vi "PathFinder.vi"(7 "All Lines":T3, 8 "Target Z":dbl format="%#_13g", 9 "Target X":dbl format="%#_13g", 11 "Posit Array":T1[](array[typedef])) -> (0 "Same Line +Dir?":bool, 1 "Path Found?":bool, 2 "Next Pos":cluster{"Line Index":i32, "Line Pos Index ":i32}, 3 "Shortest Path":T2[](array[typedef]), 4 "Index on Line":i32)   [LabVIEW 2014, in "Map Data.lvlib"]
uses:
  Map Data.lvlib
  All-Lines.ctl
  LineCluster.ctl
  LineConnection.ctl
  Components/PathFinder/Controls/PathControl.ctl
  Contact Data/Position.ctl
  Contact Data/Contact Data.lvlib
panel:
  out "All Distances":i32[](array[numeric])
  out "Distance (Points)":i32
  out "Path taken out":T2[][](array[typedef])
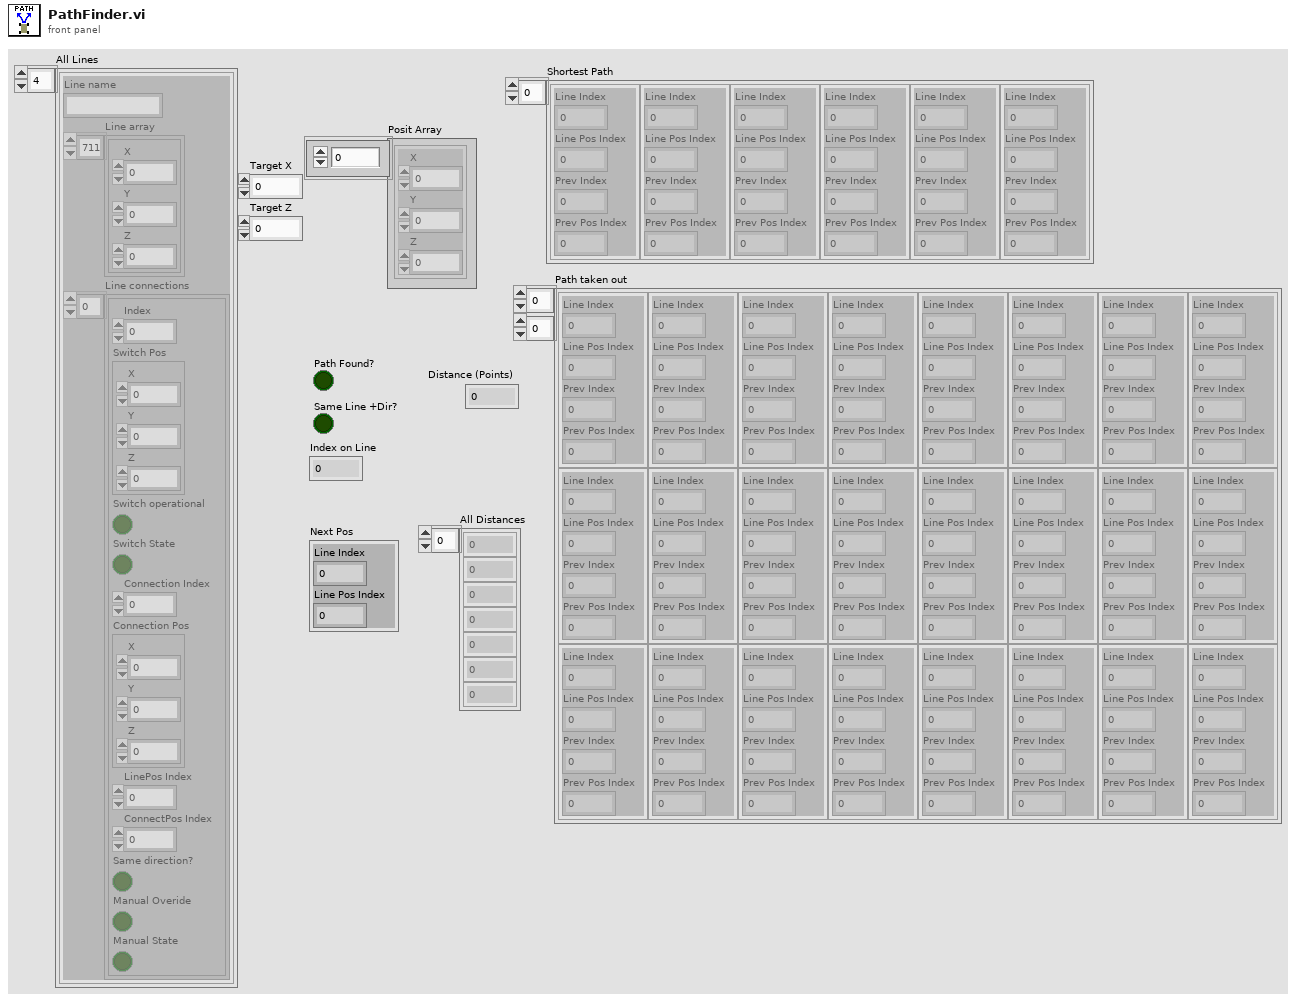
[diagram p1: front panel]
types:
  T1 = typedef "Contact Data.lvlib/Position.ctl" = cluster{"X":dbl, "Y":dbl, "Z":dbl}
  T2 = typedef "PathControl.ctl" = cluster{"Line Index":i32, "Line Pos Index ":i32, "Prev Index ":i32, "Prev Pos Index":i32}
  T3 = typedef "Map Data.lvlib/All-Lines.ctl" = T4[]
  T4 = typedef "Map Data.lvlib/LineCluster.ctl" = cluster{"Line name":string, "Line array":cluster{"X":dbl, "Y":dbl, "Z":dbl}[], "Line connections":T5[]}
  T5 = typedef "LineConnection.ctl" = cluster{"Index":i32, "Switch Pos":cluster{"X":dbl, "Y":dbl, "Z":dbl}, "Switch operational":bool, "Switch State":bool, "Connection Index":i32, "Connection Pos":cluster{"X":dbl, "Y":dbl, "Z":dbl}, "LinePos Index":i32, "ConnectPos Index":i32, "Same direction?":bool, "Manual Overide":bool, "Manual State":bool}
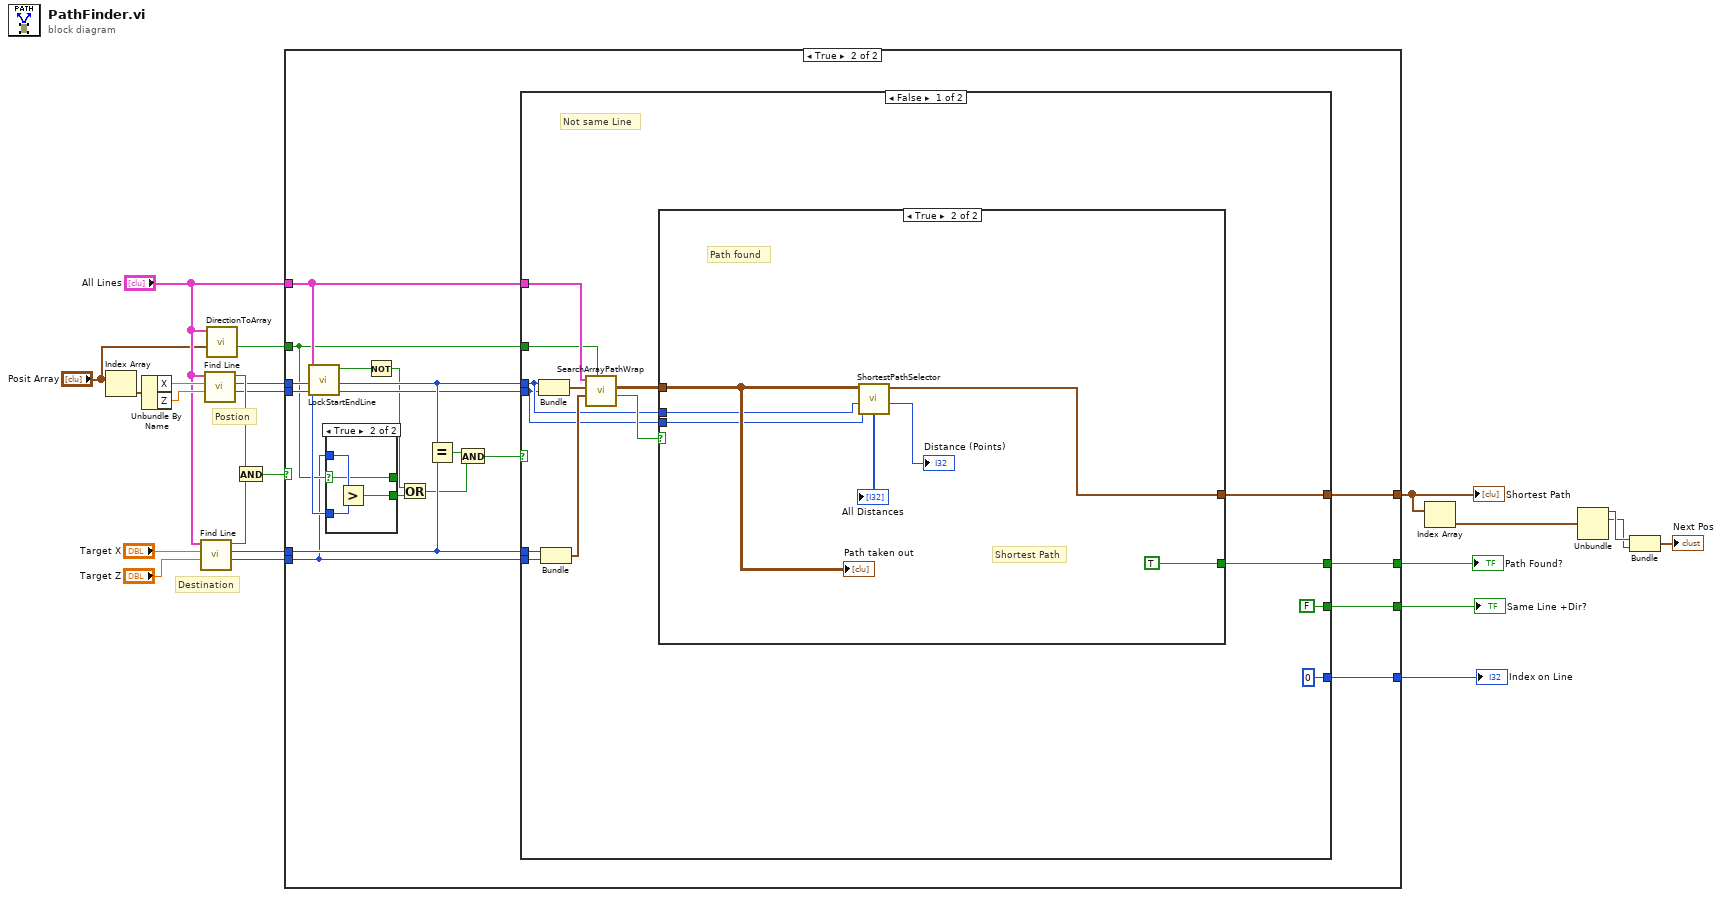
[diagram p0: block diagram]
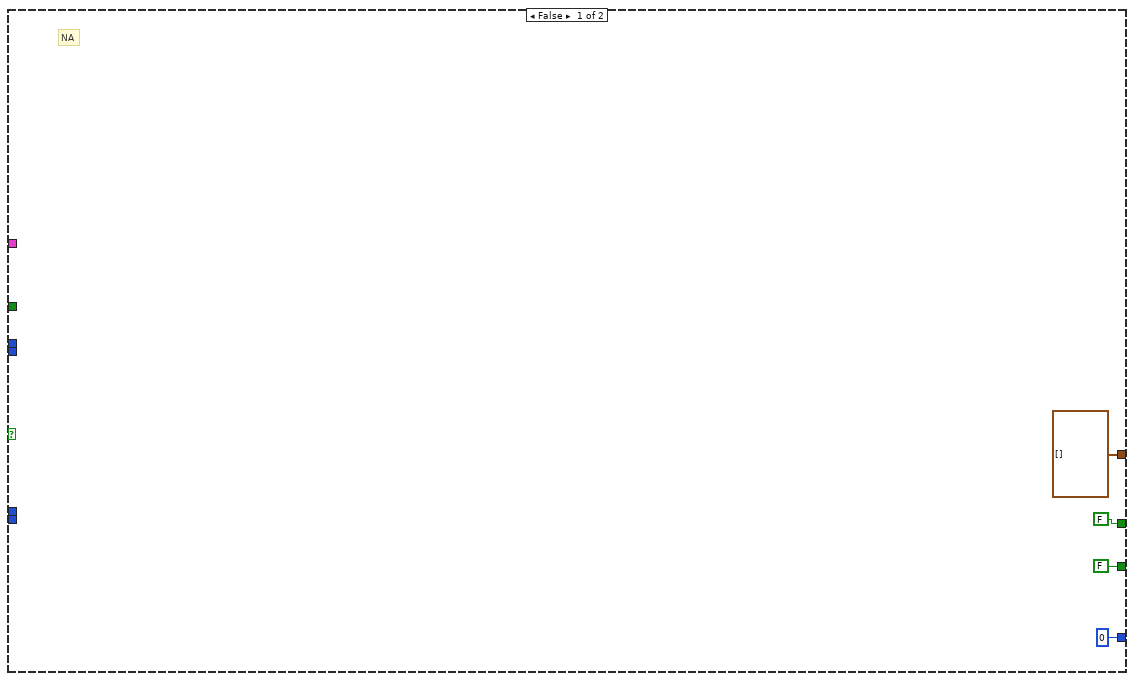
[diagram p2: hidden frame]
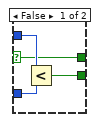
[diagram p3: hidden frame]
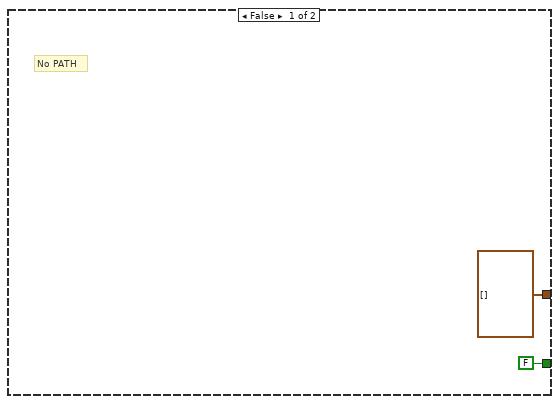
[diagram p4: hidden frame]
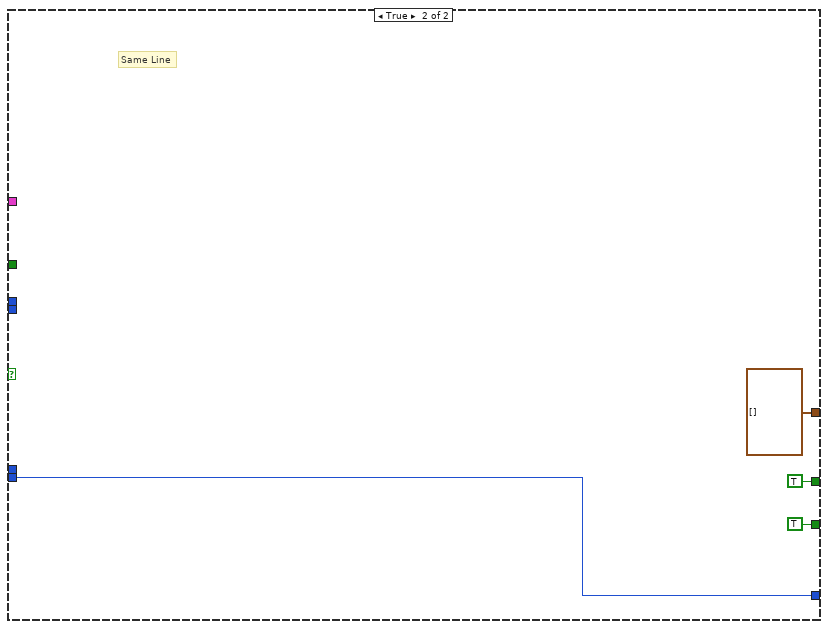
[diagram p5: hidden frame]
diagram:
  # "Postion"
  # "Destination"
  n1 = Index Array(array="Posit Array") -> (element=w10:T1)  [unwired: 1 in]
  n2 = Unbundle By Name(w10) -> ("X"=w9:dbl, "Z"=w8:dbl)
  n3 = call "Find Line.vi"("Z"="Target Z", "X"="Target X", "All Lines"="All Lines") -> ("Index on Line"=w15:i32, "Nearest Line"=w16:i32, "Line found?"=w21:bool)  [unwired: 5 in, 1 out]
  n4 = call "Find Line.vi"("Z"=w8, "X"=w9, "All Lines"="All Lines") -> ("Index on Line"=w17:i32, "Nearest Line"=w18:i32, "Line found?"=w20:bool)  [unwired: 5 in, 1 out]
  n5 = call "DirectionToArray.vi"("Posit Array"="Posit Array", "All Lines"="All Lines") -> ("Same Dir as array?"=w5:bool)  [unwired: 9 in]
  n6 = And(x=w20, y=w21) -> (x .and. y?=w19:bool)
  n7 = case shown="True" w19 {
    tunnel: "All Lines" -> [_ w38]
    tunnel: w18 -> [_ w39]
    tunnel: w17 -> [_ w37]
    tunnel: w16 -> [_ w36]
    tunnel: w15 -> [_ w28]
    tunnel: [T2[] [] ("Path taken out") w43] -> w12
    tunnel: [FALSE w42] -> w14
    tunnel: [FALSE w41] -> w13
    tunnel: [0 ("Index on Line") w40] -> w11
    tunnel: w5 -> [_ w29]
    frame False {
      # "NA"
    }
    frame True {
      n8 = call "LockStartEndLine.vi"("index"=w39, "All Lines"=w38) -> ("Not Locked?"=w34:bool)  [unwired: 9 in]
      n9 = case shown="True" w29 {
        selector: w29 -> [w44 w48]
        tunnel: w28 -> [w47 w51]
        tunnel: w37 -> [w46 w50]
        tunnel: [w45 w49] -> w35
        tunnel: [w44 w48] -> _
        frame False {
          n10 = Less?(x=w47, y=w46) -> (x < y?=w45:bool)
        }
        frame True {
          n11 = Greater?(x=w51, y=w50) -> (0:w49:bool)
        }
      }
      n12 = Not(x=w34) -> (.not. x?=w33:bool)
      n13 = Or(x=w33, y=w35) -> (x .or. y?=w30:bool)
      n14 = Equal?(x=w39, y=w36) -> (x = y?=w31:bool)
      n15 = And(x=w31, y=w30) -> (x .and. y?=w32:bool)
      n16 = case shown="False" w32 {
        tunnel: w38 -> [w65 _]
        tunnel: w36 -> [w58 _]
        tunnel: w39 -> [w53 _]
        tunnel: [w62 T2[] [] ("Path taken out")] -> w43
        tunnel: [w61 TRUE] -> w42
        tunnel: [FALSE TRUE] -> w41
        tunnel: w28 -> [w57 w76]
        tunnel: [0 ("Index on Line") w76] -> w40
        tunnel: w37 -> [w52 _]
        tunnel: w29 -> [w54 _]
        frame False {
          # "Not same Line"
          n17 = Bundle("Nearest Line"=w53, "Index on Line"=w52) -> (w55:cluster{"Nearest Line":i32, "Index on Line":i32})  [unwired: 1 in]
          n18 = Bundle("Nearest Line"=w58, "Index on Line"=w57) -> (w56:cluster{"Nearest Line":i32, "Index on Line":i32})  [unwired: 1 in]
          n19 = call "SearchArrayPathWrap.vi"("Current Direction (T=Positive)"=w54, "Target"=w56, "Current Pos"=w55, "All Lines"=w65) -> ("Found Path?"=w64:bool, "Path taken out"=w63:T2[][])  [unwired: 6 in]
          n20 = case shown="True" w64 {
            tunnel: w63 -> [_ w73]
            tunnel: [T2[] [] ("Path taken out") w72] -> w62
            tunnel: [FALSE TRUE] -> w61
            tunnel: w53 -> [_ w70]
            tunnel: w52 -> [_ w69]
            frame False {
              # "No PATH"
            }
            frame True {
              # "Path found"
              # "Shortest Path"
              n21 = call "ShortestPathSelector.vi"("Start Pos Index"=w69, "Start Index"=w70, "Path taken in"=w73) -> ("Distance (Points)"=→"Distance (Points)":i32, "Shortest Path"=w72:T2[], "All Distances"=→"All Distances":i32[])  [unwired: 6 in]
              "Path taken out" <- w73
            }
          }
        }
        frame True {
          # "Same Line"
        }
      }
    }
  }
  "Path Found?" <- w14
  "Same Line +Dir?" <- w13
  "Index on Line" <- w11
  "Shortest Path" <- w12
  n22 = Index Array(array=w12) -> (element=w1:T2)  [unwired: 1 in]
  n23 = Unbundle(w1) -> ("Line Index"=w4:i32, "Line Pos Index"=w3:i32)  [unwired: 2 out]
  n24 = Bundle("Line Index"=w4, "Line Pos Index"=w3) -> (→"Next Pos":cluster{"Line Index":i32, "Line Pos Index ":i32})  [unwired: 1 in]
